vi "Capture@FindCircle(InOut)__Parameter.vi"(1 "ParamterIn":string) -> (0 "ParamterOut":string)   [LabVIEW 2020]
panel:
  in  "Point":string(combo)
  in  "CamName":string(combo)
  in  "Confirm":bool
  # "Capture@FindCircle/Edge/Gap/Point $Capture,$Point"
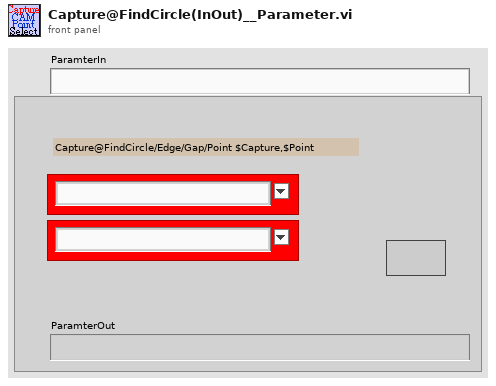
[diagram p1: front panel]
types:
  T1 = enum16{"Get", "UpdatePointS", "Init", "UpdateIndex", "GetCurrent&Index+1", "GetWithIndex", "ChkLast", "GetCurrent"}
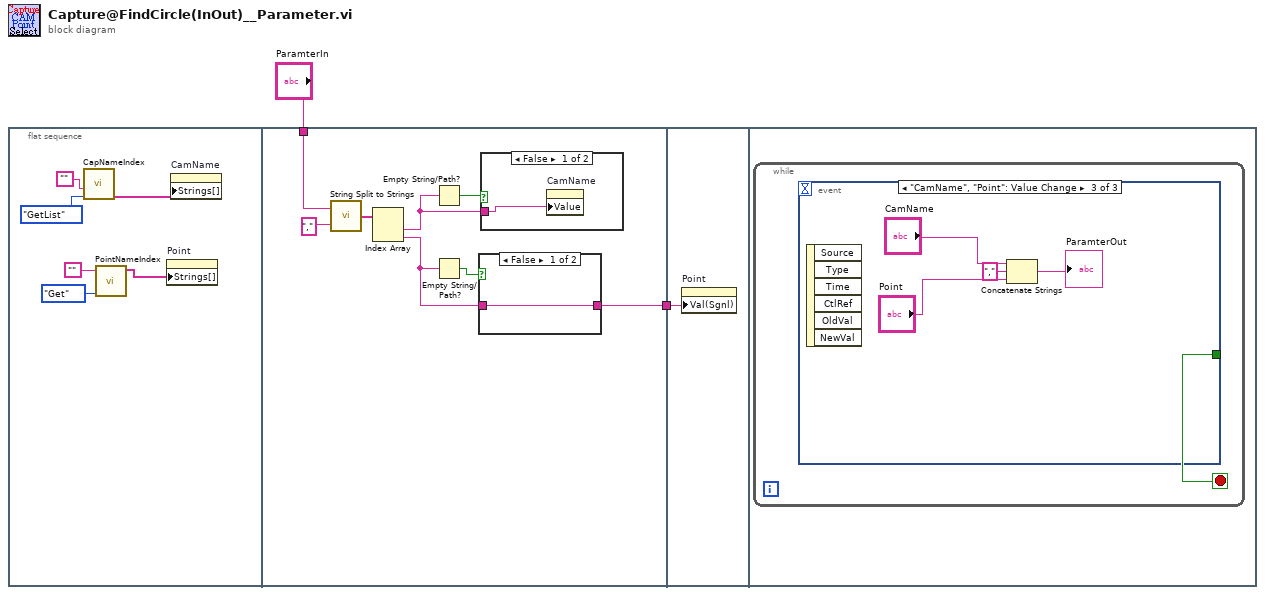
[diagram p0: block diagram]
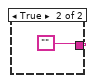
[diagram p2: hidden frame]
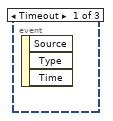
[diagram p4: hidden frame]
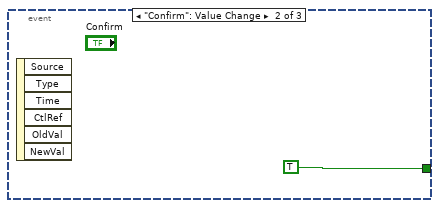
[diagram p5: hidden frame]
diagram:
  n1 = flat-sequence {
    tunnel: "ParamterIn" -> [w14]
    tunnel: [w9] -> w1
    tunnel: w1 -> [w20]
    frame #0 {
      n2 = call "CapNameIndex.vi"("OP"=enum16{"AddCam", "GetIndex", "Init", "GetList"}."GetList", "CamName"="") -> ("DeviceList"=w7:string[])  [unwired: 2 in, 3 out]
      n3 = call "PointNameIndex.vi"("OP"=T1."Get", "PointName"="") -> ("PointNameList"=w3:string[])  [unwired: 4 in, 5 out]
      n4 = property on="Point" class="CmbBox"("Strings[]"=w3) -> ()  [unwired: 2 in, 2 out]
      n5 = property on="CamName" class="CmbBox"("Strings[]"=w7) -> ()  [unwired: 2 in, 2 out]
    }
    frame #1 {
      n6 = call "String Split to Strings.vi"("search string/char (-)"=",", "String"=w14) -> ("Array"=w16:string[])
      n7 = Index Array(array=w16) -> (element #1=w12:string, element #2=w10:string)  [unwired: 2 in]
      n8 = Empty String/Path?(string/path=w12) -> (empty?=w13:bool)
      n9 = Empty String/Path?(string/path=w10) -> (empty?=w11:bool)
      n10 = case shown="False" w11 {
        tunnel: [w17 ""] -> w9
        tunnel: w10 -> [w17 _]
        frame False {
        }
        frame True {
        }
      }
      n11 = case shown="False" w13 {
        tunnel: w12 -> [w19 _]
        frame False {
          n12 = property on="CamName" class="CmbBox"("Value"=w19) -> ()  [unwired: 2 in, 2 out]
        }
        frame True {
        }
      }
    }
    frame #2 {
      n13 = property on="Point" class="CmbBox"("Val(Sgnl)"=w20) -> ()  [unwired: 2 in, 2 out]
    }
    frame #3 {
      n14 = while {
        stop <- w21 stop-if-true
        n15 = event shown="[2] \"CamName\", \"Point\": Value Change" {
          selector: _ -> [_ _ _]
          dyn-events: _ -> [_ _ _]
          timeout: _ -> [_ _ _]
          tunnel: [_ TRUE _] -> w21
          event Timeout {
            n16 = event-data() -> ()  [unwired: 1 in, 3 out]
          }
          event "Confirm": Value Change {
            n17 = event-data() -> ()  [unwired: 1 in, 6 out]
          }
          event "CamName", "Point": Value Change {
            n18 = event-data() -> ()  [unwired: 1 in, 6 out]
            n19 = Concatenate Strings("CamName", "," ("string"), "Point") -> (→"ParamterOut":string)
          }
        }
      }
    }
  }
